vi "Frequencies.vi"(7 "Mp":dbl, 8 "RPM":dbl, 9 "Nr":dbl, 10 "Np":dbl, 11 "Ns":dbl) -> (3 "char freqs":T1)   [LabVIEW 2021]
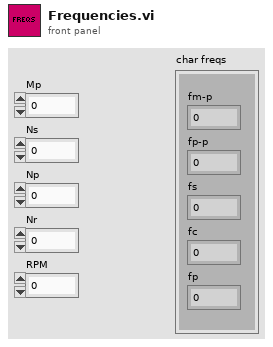
[diagram p1: front panel]
types:
  T1 = cluster{"fm-p":dbl, "fp-p":dbl, "fs":dbl, "fc":dbl, "fp":dbl}
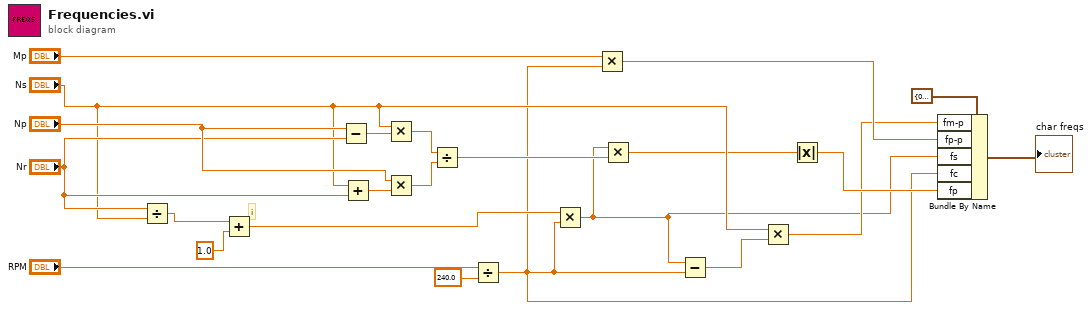
[diagram p0: block diagram]
diagram:
  # "i"
  n1 = Divide(x="Nr", y="Ns") -> (x/y=w10:dbl)
  n2 = Add(x=w10, y=1.0) -> (x+y=w9:dbl)
  n3 = Subtract(x="Np", y="Nr") -> (x-y=w20:dbl)
  n4 = Add(x="Ns", y="Nr") -> (x+y=w21:dbl)
  n5 = Multiply(x="Ns", y=w20) -> (x*y=w19:dbl)
  n6 = Multiply(x="Np", y=w21) -> (x*y=w18:dbl)
  n7 = Divide(x=w19, y=w18) -> (x/y=w17:dbl)
  n8 = Divide(x="RPM", y=240.0) -> (x/y=w3:dbl)
  n9 = Multiply(x=w9, y=w3) -> (x*y=w2:dbl)
  n10 = Multiply(x="Mp", y=w3) -> (x*y=w5:dbl)
  n11 = Multiply(x=w2, y=w17) -> (x*y=w8:dbl)
  n12 = Subtract(x=w2, y=w3) -> (x-y=w22:dbl)
  n13 = Multiply(x="Ns", y=w22) -> (x*y=w4:dbl)
  n14 = Absolute Value(x=w8) -> (abs(x)=w6:dbl)
  n15 = Bundle By Name(cluster=T1 {"fm-p"=0.0, "fp-p"=0.0, "fs"=0.0, "fc"=0.0, "fp"=0.0} ("char freqs 2"), "fm-p"=w4, "fp-p"=w5, "fs"=w2, "fc"=w3, "fp"=w6) -> (→"char freqs":T1)
